vi "Comprar.vi"(8 "error in (no error)":errorcluster, 10 "Pagar":bool, 11 "coffee Actor in":refnum<class "coffee Actor.lvclass">) -> (0 "error out":errorcluster, 3 "coffee Actor out":refnum<class "coffee Actor.lvclass">)   [LabVIEW 2019, in "coffee Actor.lvlib" / "coffee Actor.lvclass"]
uses:
  coffee Actor.lvclass
  C:/Program Files (x86)/National Instruments/LabVIEW 2019/vi.lib/ActorFramework/Actor/Actor.lvclass
  <vilib>/ActorFramework/Actor/Actor.lvclass/Actor.ctl
  coffee Actor.lvclass/coffee Actor.ctl
  UI Actor Messages/comprarcafe Msg/comprarcafe Msg.lvclass/comprarcafe Msg.ctl
  <vilib>/ActorFramework/Message Enqueuer/Message Enqueuer.lvclass/Message Enqueuer.ctl
  <vilib>/ActorFramework/Message Enqueuer/Enqueue.vi
  UI Actor Messages/comprarcafe Msg/comprarcafe Msg.lvclass
  C:/Program Files (x86)/National Instruments/LabVIEW 2019/vi.lib/ActorFramework/Message/Message.lvclass
  <vilib>/ActorFramework/Message Priority Queue/Priority Enqueue.vi
  <vilib>/ActorFramework/Actor/Actor.lvclass
panel:
  in  "Cluster":T1
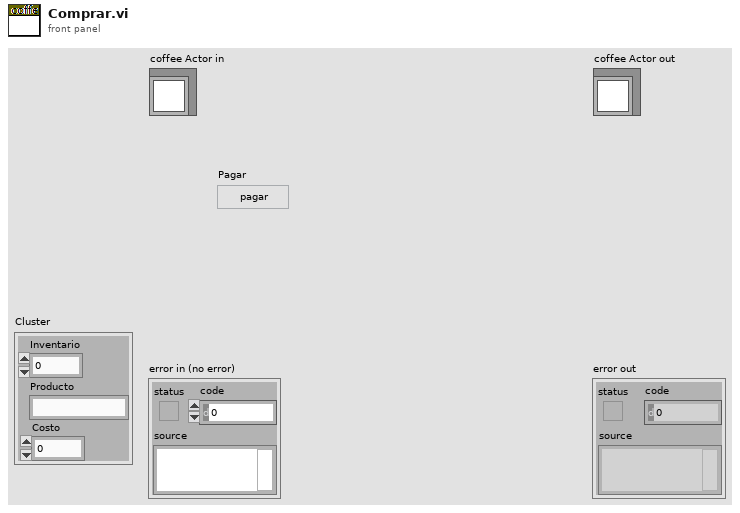
[diagram p1: front panel]
types:
  T1 = cluster{"Inventario":i32, "Producto":string, "Costo":dbl}
  T2 = cluster{"ListaSelect[0]":string, "ListaSelect[1]":string, "ListaSelect[2]":string, "ListaSelect[3]":string, "ListaSelect[4]":string, "ListaSelect[5]":string, "ListaSelect[6]":string, "ListaSelect[7]":string, "ListaSelect[8]":string}
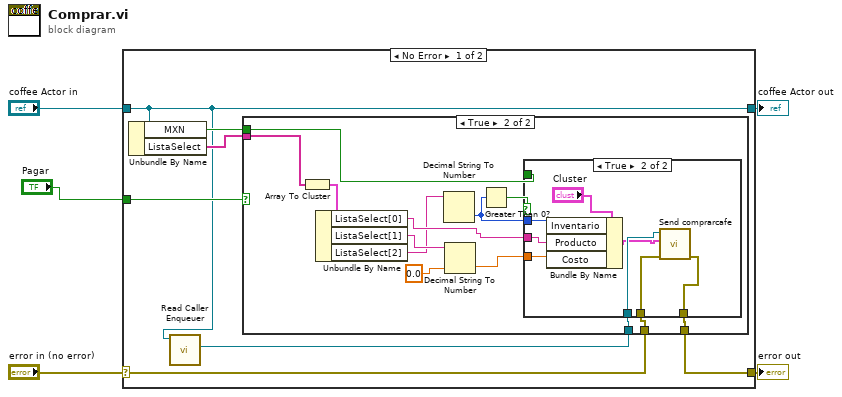
[diagram p0: block diagram]
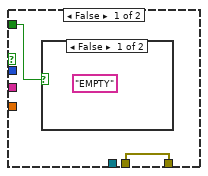
[diagram p3: hidden frame]
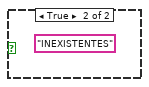
[diagram p4: hidden frame]
diagram:
  n1 = case shown="No Error" "error in (no error)" {
    selector: "error in (no error)" -> [w8 w38]
    tunnel: [w7 w38] -> w4
    tunnel: [w6 w37] -> w2
    tunnel: "coffee Actor in" -> [w6 w37]
    tunnel: "Pagar" -> [w9 _]
    frame No Error {
      n2 = Unbundle By Name(w6) -> ("MXN"=w11:bool, "ListaSelect"=w12:string[])
      n3 = call <vilib>:"Read Caller Enqueuer.vi"("Actor"=w6) -> ("Caller Enqueuer"=w10:refnum<class "Message Enqueuer.lvclass">)  [unwired: 10 in]
      n4 = case shown="True" w9 {
        tunnel: w12 -> [_ w17]
        tunnel: w11 -> [_ w25]
        tunnel: w10 -> [_ w19]
        tunnel: [w13 w18] -> w7
        tunnel: w8 -> [w13 w14]
        frame False {
        }
        frame True {
          n5 = Array To Cluster(array=w17) -> (cluster=w26:T2)
          n6 = Unbundle By Name(w26) -> ("ListaSelect[0]"=w20:string, "ListaSelect[1]"=w16:string, "ListaSelect[2]"=w15:string)
          n7 = Decimal String To Number(string=w15) -> (number=w23:i32)  [unwired: 2 in, 1 out]
          n8 = Decimal String To Number(string=w16, default (0L)=0.0) -> (number=w21:dbl)  [unwired: 1 in, 1 out]
          n9 = Greater Than 0?(x=w23) -> (x > 0?=w24:bool)
          n10 = case shown="True" w24 {
            tunnel: w25 -> [w27 _]
            tunnel: w23 -> [_ w36]
            tunnel: w21 -> [_ w34]
            tunnel: w20 -> [_ w33]
            tunnel: w19 -> [_ w32]
            tunnel: [w28 w30] -> w18
            tunnel: w14 -> [w28 w31]
            frame False {
              n11 = case shown="False" w27 {
                frame False {
                  (unwired) "EMPTY"
                }
                frame True {
                  (unwired) "INEXISTENTES"
                }
              }
            }
            frame True {
              n12 = Bundle By Name(cluster="Cluster", "Inventario"=w36, "Producto"=w33, "Costo"=w34) -> (w29:T1)
              n13 = call "Send comprarcafe.vi"("error in (no error)"=w31, "Cluster"=w29, "Message Enqueuer"=w32) -> ("error out"=w30:errorcluster)  [unwired: 7 in, 1 out]
            }
          }
        }
      }
    }
    frame Error {
    }
  }
  "error out" <- w4
  "coffee Actor out" <- w2
